vi "Script_Timing_Check_Wfm_Existence.vi"(8 "error  in":errorcluster caption="error in", 10 "SOFTWARE Inputs":T1={"Application Directory"=path "D:/S.O.F.T.S/LABVIEW/PIL", "Software Version"="1.0.0", "Data Path"=path "D:/PIRENEA/DATA", "XML Path"=path "D:/PIRENEA/DATA", "XML File Filter"="*.xml", "XML Saved Path"=path "D:/PIRENEA/DATA/SAVED", "Excit Scripts Path"=path "D:/PIRENEA/TECHNICAL/EXCIT_SCRIPTS", "Excit Scripts File Filter"="*.txt", "Excit Waveforms Path"=path "D:/PIRENEA/TECHNICAL/EXCIT_WFMS", "Excit Waveforms File Filter"="*.bin", "Timing Scripts Path"=path "D:/PIRENEA/TECHNICAL/TIMING_SCRIPTS", "Timing Scripts File Filter"="*.txt", "Timing Waveforms Path"=path "D:/PIRENEA/TECHNICAL/TIMING_WFMS", "Timing Waveforms File Filter"="*.bin", "Trapping Waveforms Path"=path "D:/PIRENEA/TECHNICAL/TRAPPING_WFMS", "Trapping Waveforms File Filter"="*.bin"}, 11 "Table of Waveforms":string[](array[string])) -> (0 "error out":errorcluster)   [LabVIEW 2018]
doc: "This VI checks if the timing waveforms required by the script are present on disk.\n\n1. The path ofr waveforms and script has to be checked before running this VI.\n2. If a waveform is missing, this VI generates an error message."
uses:
  controls/SOFTWARE_Inputs.ctl
  <vilib>/Utility/error.llb/Error Cluster From Error Code.vi
  <vilib>/ErrorRing/Error Ring.xnode
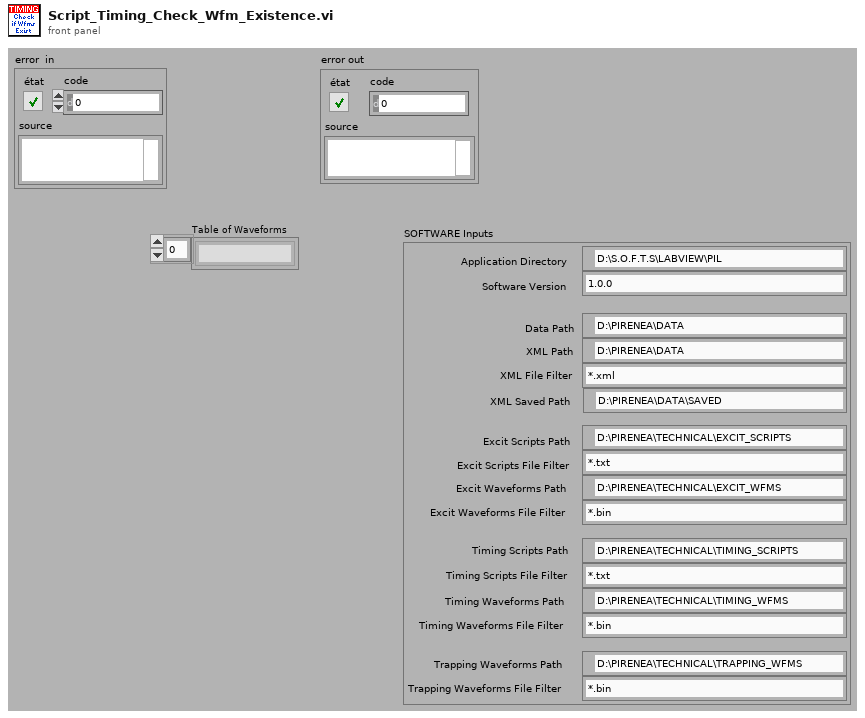
[diagram p1: front panel]
types:
  T1 = typedef "SOFTWARE_Inputs.ctl" = cluster{"Application Directory":path, "Software Version":string, "Data Path":path, "XML Path":path, "XML File Filter":string, "XML Saved Path":path, "Excit Scripts Path":path, "Excit Scripts File Filter":string, "Excit Waveforms Path":path, "Excit Waveforms File Filter":string, "Timing Scripts Path":path, "Timing Scripts File Filter":string, "Timing Waveforms Path":path, "Timing Waveforms File Filter":string, "Trapping Waveforms Path":path, "Trapping Waveforms File Filter":string}
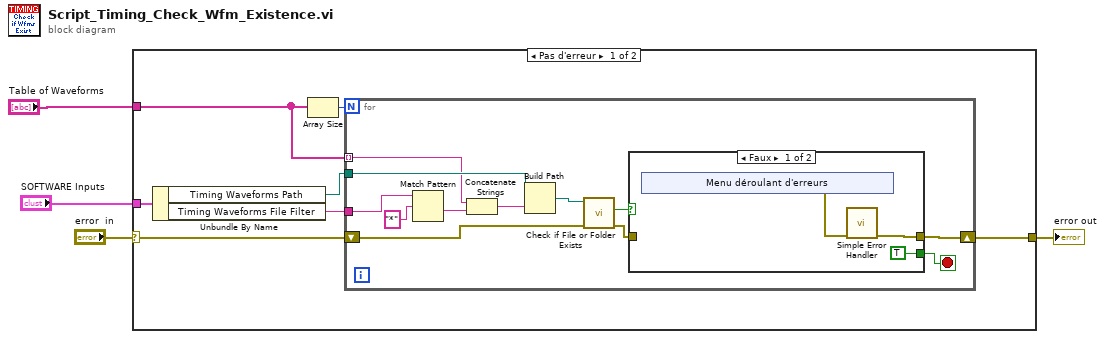
[diagram p0: block diagram]
diagram:
  n1 = case shown="Pas d'erreur" "error  in" {
    selector: "error  in" -> [w11 w33]
    tunnel: [w7 w33] -> w4
    tunnel: "SOFTWARE Inputs" -> [w10 _]
    tunnel: "Table of Waveforms" -> [w5 _]
    frame No Error {
      n2 = Unbundle By Name(w10) -> ("Timing Waveforms Path"=w9:path, "Timing Waveforms File Filter"=w8:string)
      n3 = Array Size(array=w5) -> (size(s)=w6:i32)
      n4 = for {
        N: w6 -> [_]
        tunnel: w5 -> [w19] mode=indexing
        tunnel: w9 -> [w23]
        tunnel: w8 -> [w22]
        shift-right: [w14] -> w7
        shift-left: w11 -> [w16]
        stop <- w12 stop-if-true
        n5 = Match Pattern(string=w22, regular expression="*" ("expression régulière")) -> (after substring=w20:string)  [unwired: 1 in, 3 out]
        n6 = Concatenate Strings(w19, w20) -> (w13:string)
        n7 = Build Path(base path=w23, name or relative path=w13) -> (appended path=w18:path)
        n8 = call <vilib>:"Check if File or Folder Exists.vi"("error in (no error)"=w16, "path"=w18) -> ("error out"=w15:errorcluster, "file or folder exists?"=w17:bool)  [unwired: 7 in, 1 out]
        n9 = case shown="Faux" w17 {
          tunnel: [w26 w32] -> w14
          tunnel: w15 -> [_ w32]
          tunnel: [TRUE _] -> w12
          frame False {
            n10 = xnode "Menu déroulant d'erreurs"() -> ("sortie d'erreur"=w25:errorcluster)
            n11 = call <vilib>:"Simple Error Handler.vi"("error in (no error)"=w25) -> ("error out"=w26:errorcluster)  [unwired: 4 in, 4 out]
          }
          frame True {
          }
        }
      }
    }
    frame Error {
    }
  }
  "error out" <- w4
